vi "Dax_Control_Enumerator.vi"(8 "Gain (dB) Ref":refnum<vi>, 9 "Voltage (V) Ref":refnum<vi>, 10 "Freq (MHz) Ref":refnum<vi>) -> (1 "Voltage":T1, 2 "Gain":T1, 3 "Freq":T1)   [LabVIEW 2022 SP3]
uses:
  <vilib>/Utility/miscctls.llb/LVStringsAndValuesArrayTypeDef_U16.ctl
  PulserGlobals.vi
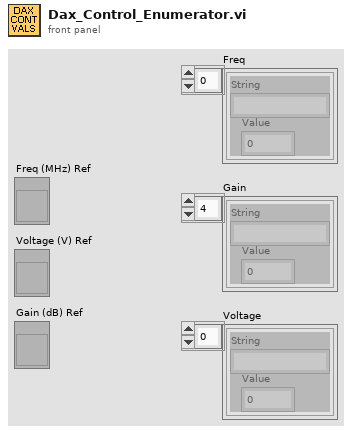
[diagram p1: front panel]
types:
  T1 = typedef "LVStringsAndValuesArrayTypeDef_U16.ctl" = cluster{"String":string, "Value":u16}[]
  T2 = typedef "Daxsonics_Pulsers.ctl" = enum16{"BP1", "BP2_A", "BP2_B", "10ERS8", "New2021"}
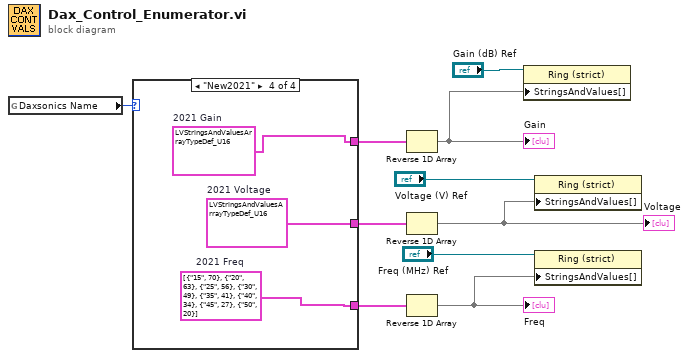
[diagram p0: block diagram]
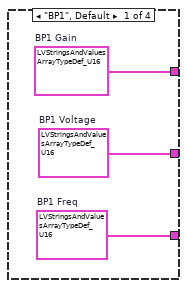
[diagram p2: hidden frame]
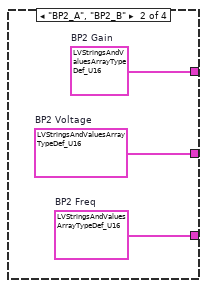
[diagram p3: hidden frame]
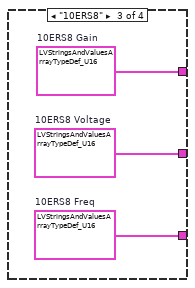
[diagram p4: hidden frame]
diagram:
  n1 = global read "PulserGlobals.vi" "Daxsonics Name"() -> (w4:T2)
  n2 = case shown="\"New2021\"" w4 {
    tunnel: [w11 w14 w19 w20] -> w3
    tunnel: [w12 w15 w18 w22] -> w2
    tunnel: [w13 w16 w17 w21] -> w1
    frame "BP1", Default {
      w12 = T1 [{"String"="0", "Value"=0}, {"String"="10", "Value"=10}, {"String"="15", "Value"=15}, {"String"="20", "Value"=20}, {"String"="25", "Value"=25}, {"String"="30", "Value"=30}, {"String"="35", "Value"=35}, {"String"="40", "Value"=40}, {"String"="45", "Value"=45}, {"String"="50", "Value"=50}, {"String"="55", "Value"=55}, {"String"="60", "Value"=60}, {"String"="65", "Value"=65}, {"String"="70", "Value"=70}, {"String"="75", "Value"=75}, {"String"="80", "Value"=80}, {"String"="85", "Value"=85}, {"String"="90", "Value"=90}, {"String"="95", "Value"=95}, {"String"="100", "Value"=100}]  # BP1 Voltage
      w11 = T1 [{"String"="0", "Value"=0}, {"String"="3", "Value"=3}, {"String"="6", "Value"=6}, {"String"="9", "Value"=9}, {"String"="12", "Value"=12}, {"String"="15", "Value"=15}, {"String"="18", "Value"=18}, {"String"="21", "Value"=21}, {"String"="24", "Value"=24}, {"String"="27", "Value"=27}, {"String"="30", "Value"=30}, {"String"="33", "Value"=33}, {"String"="36", "Value"=36}, {"String"="39", "Value"=39}, {"String"="42", "Value"=42}, {"String"="45", "Value"=45}]  # BP1 Gain
      w13 = T1 [{"String"="4", "Value"=4}, {"String"="6", "Value"=6}, {"String"="8", "Value"=8}, {"String"="10", "Value"=10}, {"String"="12", "Value"=12}, {"String"="15", "Value"=15}, {"String"="17", "Value"=17}, {"String"="20", "Value"=20}, {"String"="25", "Value"=25}, {"String"="30", "Value"=30}, {"String"="35", "Value"=35}, {"String"="40", "Value"=40}, {"String"="45", "Value"=45}, {"String"="50", "Value"=50}]  # BP1 Freq
    }
    frame "BP2_A", "BP2_B" {
      w16 = T1 [{"String"="4", "Value"=4}, {"String"="6", "Value"=6}, {"String"="8", "Value"=8}, {"String"="10", "Value"=10}, {"String"="12", "Value"=12}, {"String"="15", "Value"=15}, {"String"="17", "Value"=17}, {"String"="20", "Value"=20}, {"String"="25", "Value"=25}, {"String"="30", "Value"=30}, {"String"="35", "Value"=35}, {"String"="40", "Value"=40}, {"String"="45", "Value"=45}, {"String"="50", "Value"=50}]  # BP2 Freq
      w15 = T1 [{"String"="0", "Value"=0}, {"String"="10", "Value"=10}, {"String"="20", "Value"=20}, {"String"="30", "Value"=30}, {"String"="40", "Value"=40}, {"String"="50", "Value"=50}, {"String"="60", "Value"=60}, {"String"="70", "Value"=70}, {"String"="80", "Value"=80}, {"String"="90", "Value"=90}, {"String"="100", "Value"=100}, {"String"="110", "Value"=110}, {"String"="120", "Value"=120}, {"String"="130", "Value"=130}, {"String"="140", "Value"=140}, {"String"="150", "Value"=150}, {"String"="160", "Value"=160}, {"String"="170", "Value"=170}, {"String"="180", "Value"=180}, {"String"="190", "Value"=190}]  # BP2 Voltage
      w14 = T1 [{"String"="22", "Value"=22}, {"String"="25", "Value"=25}, {"String"="28", "Value"=28}, {"String"="31", "Value"=31}, {"String"="34", "Value"=34}, {"String"="37", "Value"=37}, {"String"="40", "Value"=40}, {"String"="43", "Value"=43}, {"String"="46", "Value"=46}, {"String"="49", "Value"=49}, {"String"="52", "Value"=52}, {"String"="55", "Value"=55}, {"String"="58", "Value"=58}, {"String"="61", "Value"=61}, {"String"="64", "Value"=64}]  # BP2 Gain
    }
    frame "10ERS8" {
      w17 = T1 [{"String"="10", "Value"=10}, {"String"="14", "Value"=14}, {"String"="16", "Value"=16}, {"String"="18", "Value"=18}, {"String"="20", "Value"=20}, {"String"="25", "Value"=25}, {"String"="30", "Value"=30}, {"String"="35", "Value"=35}, {"String"="40", "Value"=40}, {"String"="45", "Value"=45}]  # 10ERS8 Freq
      w18 = T1 [{"String"="0", "Value"=0}, {"String"="10", "Value"=10}, {"String"="20", "Value"=20}, {"String"="30", "Value"=30}, {"String"="40", "Value"=40}, {"String"="50", "Value"=50}, {"String"="60", "Value"=60}, {"String"="70", "Value"=70}, {"String"="80", "Value"=80}, {"String"="90", "Value"=90}, {"String"="100", "Value"=100}, {"String"="110", "Value"=110}]  # 10ERS8 Voltage
      w19 = T1 [{"String"="22", "Value"=22}, {"String"="25", "Value"=25}, {"String"="28", "Value"=28}, {"String"="31", "Value"=31}, {"String"="34", "Value"=34}, {"String"="37", "Value"=37}, {"String"="40", "Value"=40}, {"String"="43", "Value"=43}, {"String"="46", "Value"=46}, {"String"="49", "Value"=49}, {"String"="52", "Value"=52}, {"String"="55", "Value"=55}, {"String"="58", "Value"=58}, {"String"="61", "Value"=61}, {"String"="64", "Value"=64}, {"String"="67", "Value"=67}]  # 10ERS8 Gain
    }
    frame "New2021" {
      w20 = T1 [{"String"="16", "Value"=16}, {"String"="20", "Value"=20}, {"String"="24", "Value"=24}, {"String"="28", "Value"=28}, {"String"="32", "Value"=32}, {"String"="36", "Value"=36}, {"String"="40", "Value"=40}, {"String"="44", "Value"=44}, {"String"="48", "Value"=48}, {"String"="52", "Value"=52}, {"String"="60", "Value"=60}, {"String"="64", "Value"=64}]  # 2021 Gain
      w21 = T1 [{"String"="15", "Value"=70}, {"String"="20", "Value"=63}, {"String"="25", "Value"=56}, {"String"="30", "Value"=49}, {"String"="35", "Value"=41}, {"String"="40", "Value"=34}, {"String"="45", "Value"=27}, {"String"="50", "Value"=20}]  # 2021 Freq
      w22 = T1 [{"String"="0", "Value"=0}, {"String"="10", "Value"=10}, {"String"="20", "Value"=20}, {"String"="30", "Value"=30}, {"String"="40", "Value"=40}, {"String"="50", "Value"=50}, {"String"="60", "Value"=60}, {"String"="70", "Value"=70}, {"String"="80", "Value"=80}, {"String"="90", "Value"=90}, {"String"="100", "Value"=100}]  # 2021 Voltage
    }
  }
  n3 = Reverse 1D Array(array=w3) -> (reversed array=w5:T1)
  "Gain" <- w5
  n4 = Reverse 1D Array(array=w2) -> (reversed array=w6:T1)
  "Voltage" <- w6
  n5 = Reverse 1D Array(array=w1) -> (reversed array=w7:T1)
  "Freq" <- w7
  n6 = property class="Ring (strict)"(reference="Gain (dB) Ref", "StringsAndValues[]"=w5) -> ()  [unwired: 1 in, 2 out]
  n7 = property class="Ring (strict)"(reference="Voltage (V) Ref", "StringsAndValues[]"=w6) -> ()  [unwired: 1 in, 2 out]
  n8 = property class="Ring (strict)"(reference="Freq (MHz) Ref", "StringsAndValues[]"=w7) -> ()  [unwired: 1 in, 2 out]
